vi "PWM_For.vi"() -> ()   [LabVIEW 2019]
uses:
  <vilib>/rvi/Emulation/niFpgaGetClockAttributes.vi
  <vilib>/rvi/Emulation/niFpgaSctlEmulationGetInTimedLoop.vi
  <vilib>/rvi/Emulation/niFpgaEmulationReportErrorSimple.vi
  <vilib>/rvi/eio/common/nirviEmuTemplateMethod_errors.vi
  <vilib>/rvi/Emulation/niFpgaCriticalErrorInLSC.vi
  <vilib>/eio/EIONode/EIONode.xnode
panel:
  out "波形图表":u16(graph)
  out "x-1":u16
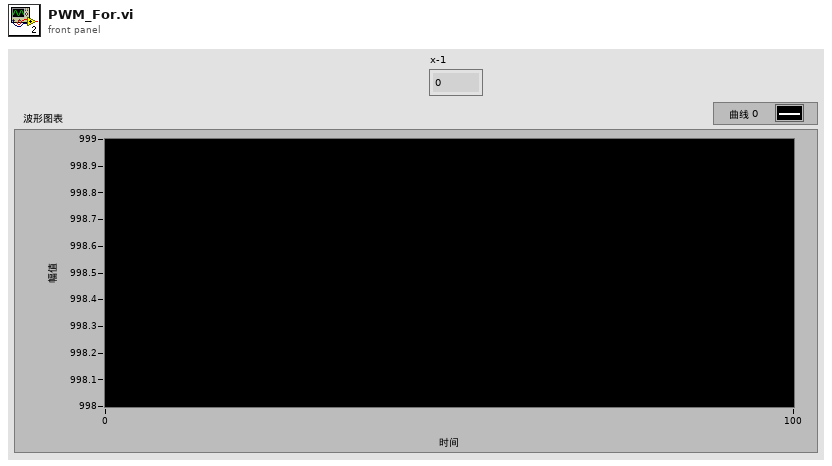
[diagram p1: front panel]
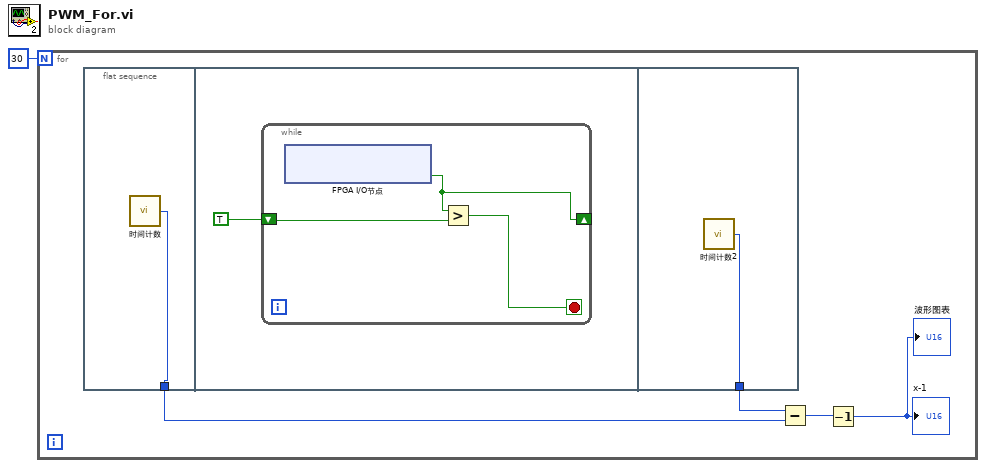
[diagram p0: block diagram]
diagram:
  n1 = for {
    N: 30 -> [_]
    n2 = flat-sequence {
      tunnel: [w6] -> w4
      tunnel: [w11] -> w5
      frame #0 {
        n3 = call "时间计数"() -> ("Tick Count(uSec)"=w6:u16)
      }
      frame #1 {
        n4 = while {
          shift-right: [w9] -> _
          shift-left: TRUE -> [w10]
          stop <- w8 stop-if-true
          n5 = xnode "FPGA I/O节点"() -> ("ConnectorB/DIO0"=w9:bool)  [unwired: 1 in, 1 out]
          n6 = Greater?(x=w9, y=w10) -> (0:w8:bool)
        }
      }
      frame #2 {
        n7 = call "时间计数2"() -> ("Tick Count(uSec)"=w11:u16)
      }
    }
    n8 = Subtract(x=w5, y=w4) -> (x-y=w3:u16)
    n9 = Decrement(x=w3) -> (x-1=→"x-1" →"波形图表":u16)
  }
